vi "gra.vi"() -> ()   [LabVIEW 2016]
doc: "projekt WIiS 201"
panel:
  in  "cluster3":T1
  in  "Cluster 2":T2
  in  "Cluster 1":T3
  out "licznik":i32[][](array[numeric])
  out "obrazy":i32[][](array[ring])
  out "emotikony":u16(ring)
  out "mat17":i32[][](array[numeric])
  out ".not. x?":bool
  out "restart":i32
  out "miny":i32
  out "flag":bool
  out "czas":dbl format="%<%M:%S>t"
  out "miny":i32[][](array[numeric])
  out "rozmiar":i32
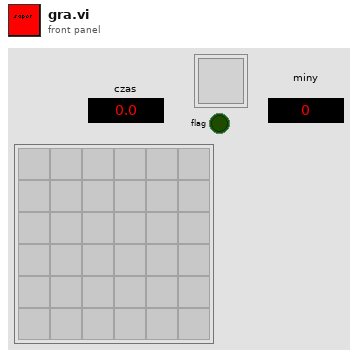
[diagram p1: front panel]
types:
  T1 = cluster{"Boolean 65":bool, "Boolean 66":bool, "Boolean 67":bool, "Boolean 68":bool, "Boolean 69":bool, "Boolean 70":bool, "Boolean 71":bool, "Boolean 72":bool, "Boolean 73":bool, "Boolean 74":bool, "Boolean 75":bool, "Boolean 76":bool, "Boolean 77":bool, "Boolean 78":bool, "Boolean 79":bool, "Boolean 80":bool, "Boolean 81":bool, "Boolean 82":bool, "Boolean 83":bool, "Boolean 84":bool, "Boolean 85":bool, "Boolean 86":bool, "Boolean 87":bool, "Boolean 88":bool, "Boolean 89":bool, "Boolean 90":bool, "Boolean 91":bool, "Boolean 92":bool, "Boolean 93":bool, "Boolean 94":bool, "Boolean 95":bool, "Boolean 96":bool, "Boolean 97":bool, "Boolean 98":bool, "Boolean 99":bool, "Boolean 100":bool, "Boolean 101":bool, "Boolean 102":bool, "Boolean 103":bool, "Boolean 104":bool, "Boolean 105":bool, "Boolean 106":bool, "Boolean 107":bool, "Boolean 108":bool, "Boolean 109":bool, "Boolean 110":bool, "Boolean 111":bool, "Boolean 112":bool, "Boolean 113":bool, "Boolean 114":bool, "Boolean 115":bool, "Boolean 116":bool, "Boolean 117":bool, "Boolean 118":bool, "Boolean 119":bool, "Boolean 120":bool, "Boolean 121":bool, "Boolean 122":bool, "Boolean 123":bool, "Boolean 124":bool, "Boolean 125":bool, "Boolean 126":bool, "Boolean 127":bool, "Boolean 128":bool, "Boolean 129":bool, "Boolean 130":bool, "Boolean 131":bool, "Boolean 132":bool, "Boolean 133":bool, "Boolean 134":bool, "Boolean 135":bool, "Boolean 136":bool, "Boolean 137":bool, "Boolean 138":bool, "Boolean 139":bool, "Boolean 140":bool, "Boolean 141":bool, "Boolean 142":bool, "Boolean 143":bool, "Boolean 144":bool, "Boolean 145":bool, "Boolean 146":bool, "Boolean 147":bool, "Boolean 148":bool, "Boolean 149":bool, "Boolean 150":bool, "Boolean 151":bool, "Boolean 152":bool, "Boolean 153":bool, "Boolean 154":bool, "Boolean 155":bool, "Boolean 156":bool, "Boolean 157":bool, "Boolean 158":bool, "Boolean 159":bool, "Boolean 160":bool, "Boolean 161":bool, "Boolean 162":bool, "Boolean 163":bool, "Boolean 164":bool, "Boolean 165":bool, "Boolean 166":bool, "Boolean 167":bool, "Boolean 168":bool, "Boolean 169":bool, "Boolean 170":bool, "Boolean 171":bool, "Boolean 172":bool, "Boolean 173":bool, "Boolean 174":bool, "Boolean 175":bool, "Boolean 176":bool, "Boolean 177":bool, "Boolean 178":bool, "Boolean 179":bool, "Boolean 180":bool, "Boolean 181":bool, "Boolean 182":bool, "Boolean 183":bool, "Boolean 184":bool, "Boolean 185":bool, "Boolean 186":bool, "Boolean 187":bool, "Boolean 188":bool, "Boolean 189":bool, "Boolean 190":bool, "Boolean 191":bool, "Boolean 192":bool, "Boolean 193":bool, "Boolean 194":bool, "Boolean 195":bool, "Boolean 196":bool, "Boolean 197":bool, "Boolean 198":bool, "Boolean 199":bool, "Boolean 200":bool, "Boolean 201":bool, "Boolean 202":bool, "Boolean 203":bool, "Boolean 204":bool, "Boolean 205":bool, "Boolean 206":bool, "Boolean 207":bool, "Boolean 208":bool}
  T2 = cluster{"Boolean 65":bool, "Boolean 66":bool, "Boolean 67":bool, "Boolean 68":bool, "Boolean 69":bool, "Boolean 70":bool, "Boolean 71":bool, "Boolean 72":bool, "Boolean 77":bool, "Boolean 78":bool, "Boolean 79":bool, "Boolean 80":bool, "Boolean 81":bool, "Boolean 82":bool, "Boolean 83":bool, "Boolean 84":bool, "Boolean 89":bool, "Boolean 90":bool, "Boolean 91":bool, "Boolean 92":bool, "Boolean 93":bool, "Boolean 94":bool, "Boolean 95":bool, "Boolean 96":bool, "Boolean 101":bool, "Boolean 102":bool, "Boolean 103":bool, "Boolean 104":bool, "Boolean 105":bool, "Boolean 106":bool, "Boolean 107":bool, "Boolean 108":bool, "Boolean 113":bool, "Boolean 114":bool, "Boolean 115":bool, "Boolean 116":bool, "Boolean 117":bool, "Boolean 118":bool, "Boolean 119":bool, "Boolean 120":bool, "Boolean 125":bool, "Boolean 126":bool, "Boolean 127":bool, "Boolean 128":bool, "Boolean 129":bool, "Boolean 130":bool, "Boolean 131":bool, "Boolean 132":bool, "Boolean 137":bool, "Boolean 138":bool, "Boolean 139":bool, "Boolean 140":bool, "Boolean 141":bool, "Boolean 142":bool, "Boolean 143":bool, "Boolean 144":bool, "Boolean 149":bool, "Boolean 150":bool, "Boolean 151":bool, "Boolean 152":bool, "Boolean 153":bool, "Boolean 154":bool, "Boolean 155":bool, "Boolean 156":bool}
  T3 = cluster{"Boolean 65":bool, "Boolean 66":bool, "Boolean 67":bool, "Boolean 68":bool, "Boolean 69":bool, "Boolean 70":bool, "Boolean 77":bool, "Boolean 78":bool, "Boolean 79":bool, "Boolean 80":bool, "Boolean 81":bool, "Boolean 82":bool, "Boolean 89":bool, "Boolean 90":bool, "Boolean 91":bool, "Boolean 92":bool, "Boolean 93":bool, "Boolean 94":bool, "Boolean 101":bool, "Boolean 102":bool, "Boolean 103":bool, "Boolean 104":bool, "Boolean 105":bool, "Boolean 106":bool, "Boolean 113":bool, "Boolean 114":bool, "Boolean 115":bool, "Boolean 116":bool, "Boolean 117":bool, "Boolean 118":bool, "Boolean 125":bool, "Boolean 126":bool, "Boolean 127":bool, "Boolean 128":bool, "Boolean 129":bool, "Boolean 130":bool}
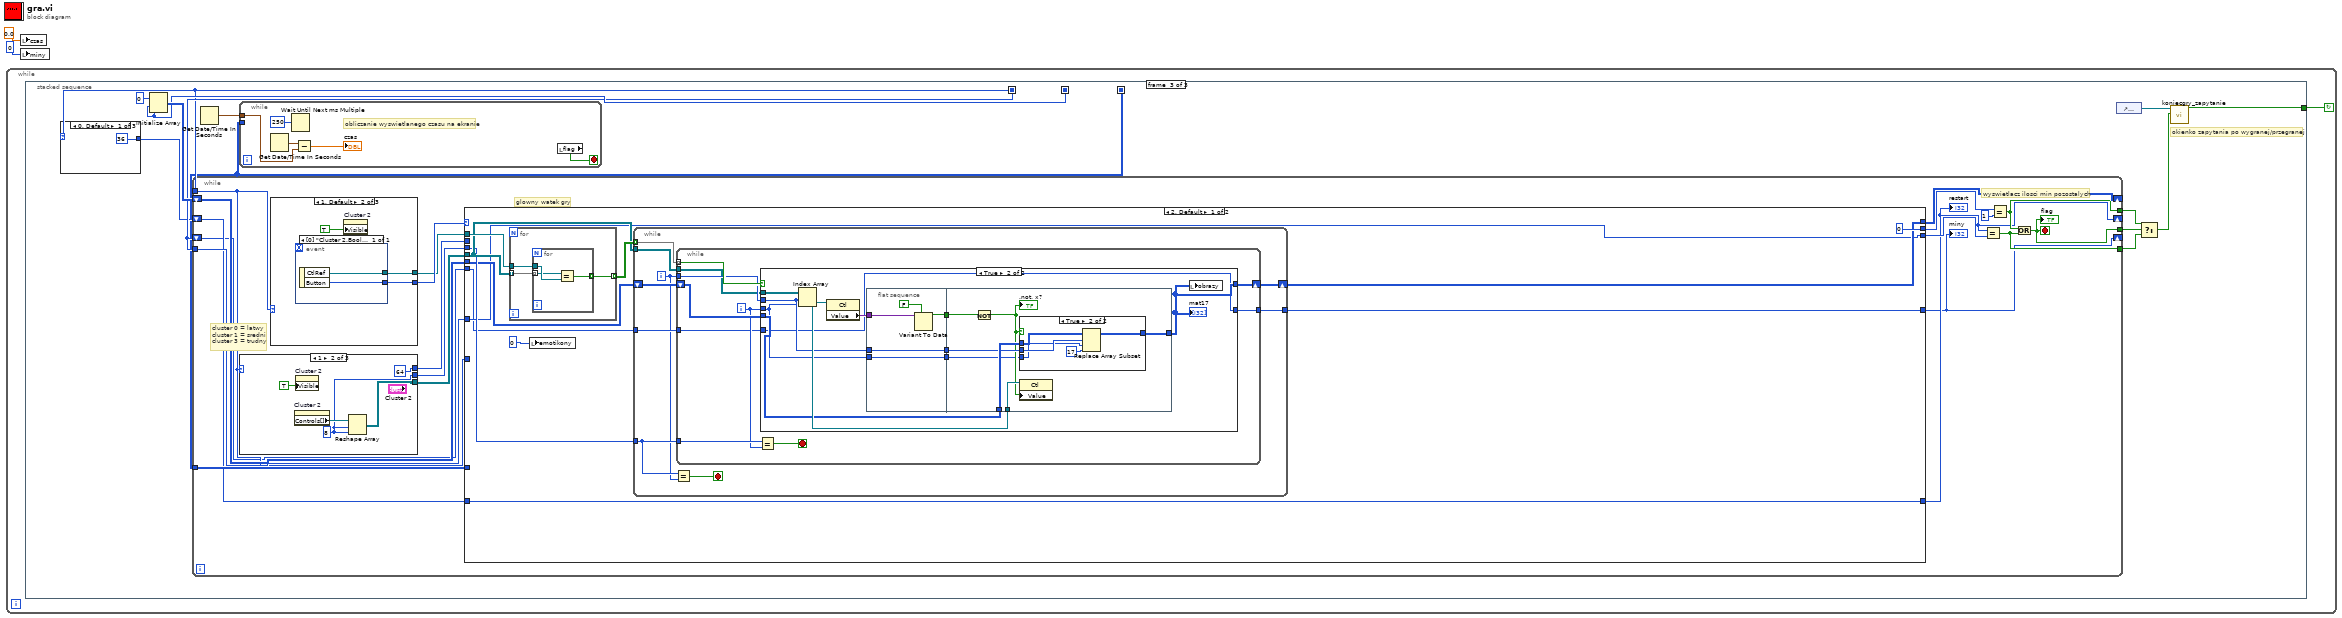
[diagram p0: block diagram]
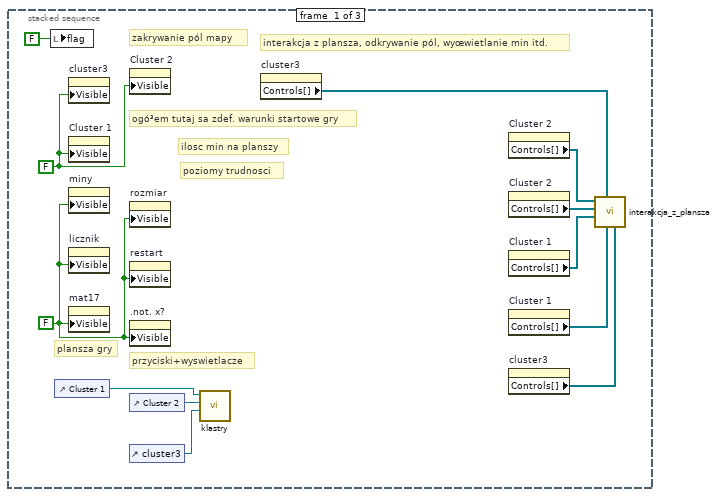
[diagram p2: hidden frame]
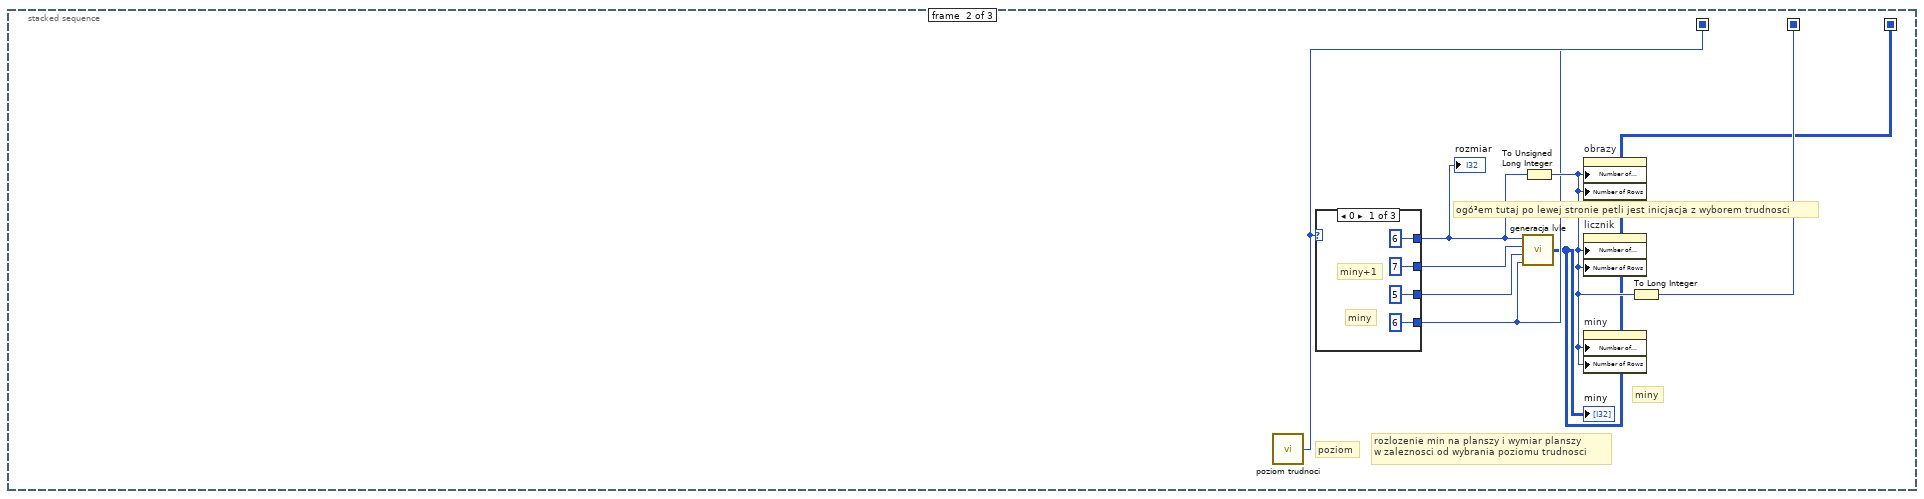
[diagram p3: hidden frame]
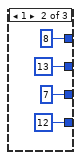
[diagram p4: hidden frame]
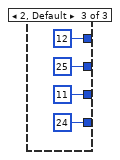
[diagram p5: hidden frame]
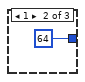
[diagram p6: hidden frame]
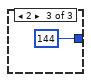
[diagram p7: hidden frame]
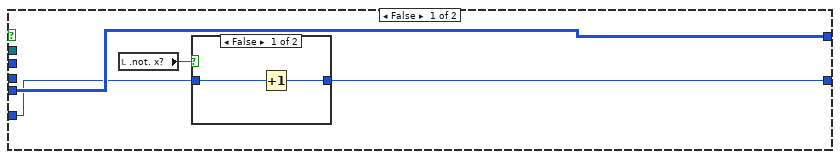
[diagram p8: hidden frame]
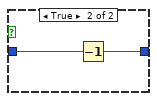
[diagram p9: hidden frame]
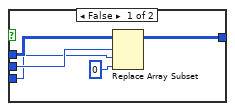
[diagram p10: hidden frame]
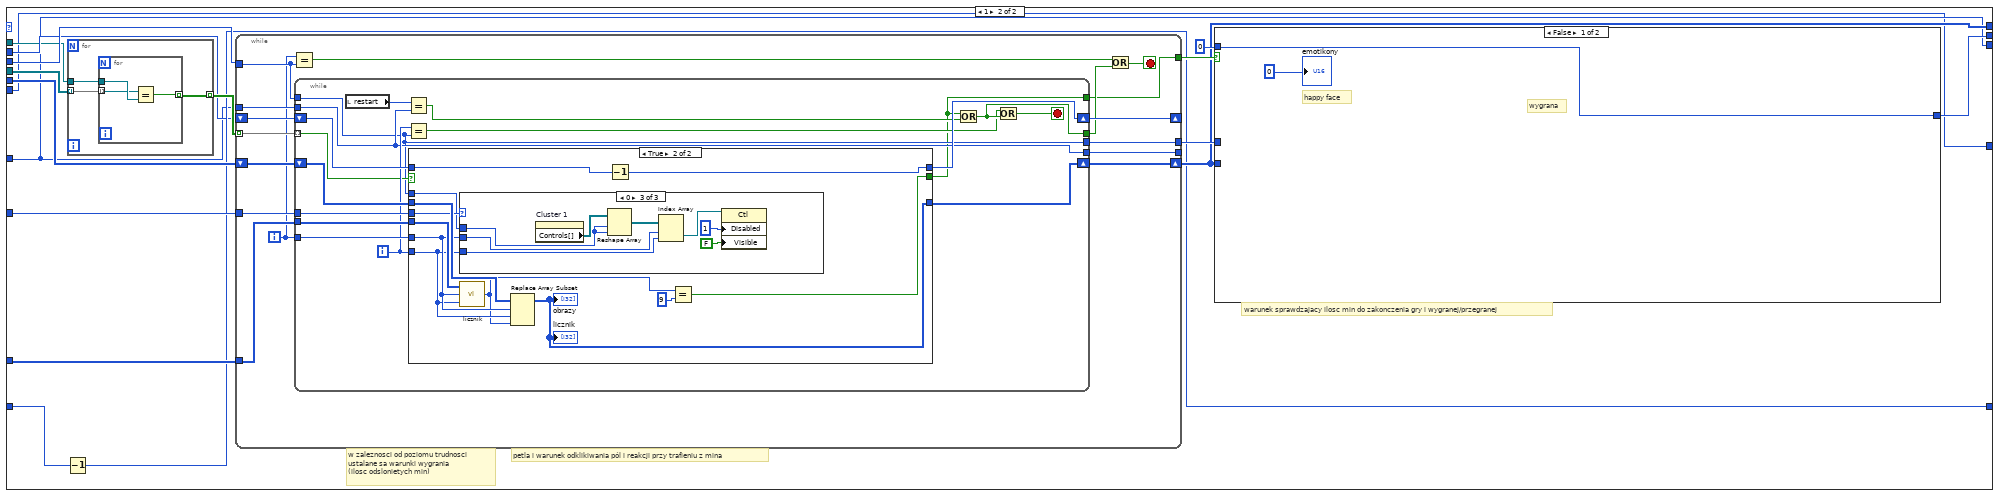
[diagram p11: hidden frame]
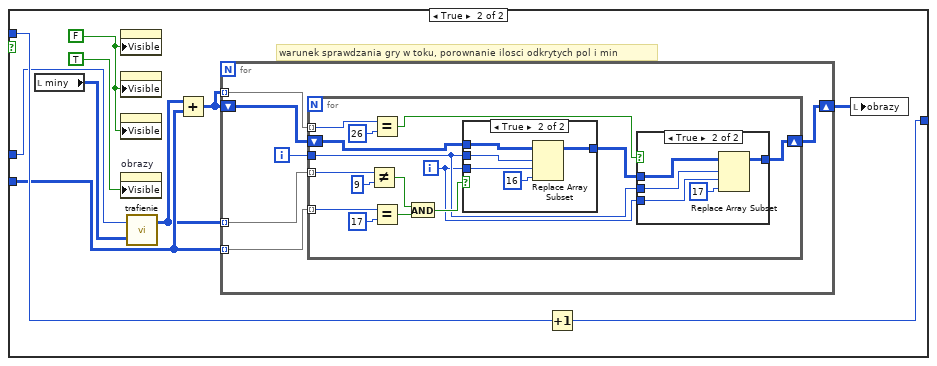
[diagram p12: hidden frame]
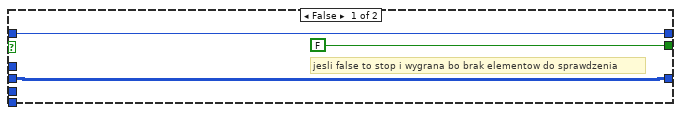
[diagram p15: hidden frame]
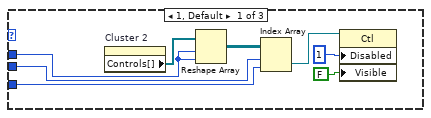
[diagram p16: hidden frame]
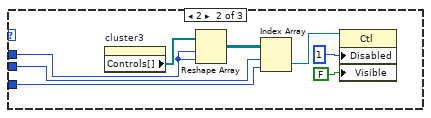
[diagram p17: hidden frame]
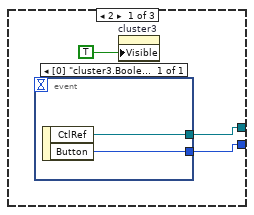
[diagram p18: hidden frame]
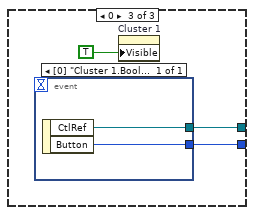
[diagram p19: hidden frame]
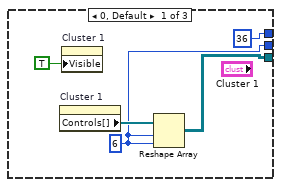
[diagram p20: hidden frame]
diagram:
  n1 = while {
    stop <- w3 continue-if-true
    n2 = stacked-sequence {
      seq-local: [_ w22 _] -> [_ _ w47]
      seq-local: [_ w16 _] -> [_ _ w37]
      seq-local: [_ w20 _] -> [_ _ w43]
      seq-local: [_ w21 _] -> [_ _ w41]
      tunnel: [_ _ w40] -> w3
      frame #0 {
        w8 = FALSE ("Visible")
        w10 = FALSE ("Visible")
        # "przyciski+wyswietlacze"
        # "interakcja z plansza, odkrywanie pól, wyœwietlanie min itd."
        # "ogó³em tutaj sa zdef. warunki startowe gry"
        # "plansza gry"
        # "zakrywanie pól mapy"
        # "ilosc min na planszy"
        # "poziomy trudnosci"
        n3 = local write "flag"(FALSE ("flag")) -> ()
        n4 = control-ref of="Cluster 1"() -> (w6:refnum<vi>)
        n5 = property on="cluster3" class="Clust (strict)"("Visible"=w10) -> ()  [unwired: 2 in, 2 out]
        n6 = property on="Cluster 1" class="Clust (strict)"("Visible"=w10) -> ()  [unwired: 2 in, 2 out]
        n7 = property on="miny" class="Arr (strict)"("Visible"=w8) -> ()  [unwired: 2 in, 2 out]
        n8 = property on="licznik" class="Arr (strict)"("Visible"=w8) -> ()  [unwired: 2 in, 2 out]
        n9 = property on="mat17" class="Arr (strict)"("Visible"=w8) -> ()  [unwired: 2 in, 2 out]
        n10 = property on="Cluster 2" class="Clust (strict)"("Visible"=w10) -> ()  [unwired: 2 in, 2 out]
        n11 = property on="rozmiar" class="DigNum (strict)"("Visible"=w8) -> ()  [unwired: 2 in, 2 out]
        n12 = property on="restart" class="DigNum (strict)"("Visible"=w8) -> ()  [unwired: 2 in, 2 out]
        n13 = property on=".not. x?" class="Bool (strict)"("Visible"=w8) -> ()  [unwired: 2 in, 2 out]
        n14 = control-ref of="Cluster 2"() -> (w5:refnum<vi>)
        n15 = control-ref of="cluster3"() -> (w4:refnum<vi>)
        n16 = call "klastry.vi"("reference 3"=w4, "reference in"=w5, "Cluster in"=w6) -> ()  [unwired: 9 in]
        n17 = property on="cluster3" class="Clust (strict)"() -> ("Controls[]"=w12:refnum<vi>[])  [unwired: 2 in, 2 out]
        n18 = property on="Cluster 2" class="Clust (strict)"() -> ("Controls[]"=w14:refnum<vi>[])  [unwired: 2 in, 2 out]
        n19 = property on="Cluster 2" class="Clust (strict)"() -> ("Controls[]"=w11:refnum<vi>[])  [unwired: 2 in, 2 out]
        n20 = property on="Cluster 1" class="Clust (strict)"() -> ("Controls[]"=w9:refnum<vi>[])  [unwired: 2 in, 2 out]
        n21 = property on="Cluster 1" class="Clust (strict)"() -> ("Controls[]"=w15:refnum<vi>[])  [unwired: 2 in, 2 out]
        n22 = property on="cluster3" class="Clust (strict)"() -> ("Controls[]"=w13:refnum<vi>[])  [unwired: 2 in, 2 out]
        n23 = call "interakcja_z_plansza.vi"("Controls[] 4"=w13, "Controls[] 6"=w15, "Controls[] 3"=w12, "Controls[]"=w9, "Controls[] 2"=w11, "Controls[] 5"=w14) -> ()  [unwired: 6 in]
      }
      frame #1 {
        # "ogó³em tutaj po lewej stronie petli jest inicjacja z wyborem trudnosci"
        # "miny"
        # "poziom"
        # "rozlozenie min na planszy i wymiar planszy \nw zaleznosci od wybrania poziomu trudnosci"
        n24 = call "poziom trudnoci.vi"() -> ("wynik wyboru"=w21:i32)
        n25 = case shown="0" w21 {
          tunnel: [6 8 12] -> w17
          tunnel: [7 13 25] -> w18
          tunnel: [6 12 24] -> w20
          tunnel: [5 7 11] -> w19
          frame 0 {
            # "miny"
            # "miny+1"
          }
          frame 1 {
          }
          frame 2, Default {
          }
        }
        "rozmiar" <- w17
        n26 = call "generacja lvle.vi"("miny"=w20, "const"=w19, "Miny+1"=w18, "rozmiar"=w17) -> ("Array"=w16:i32[][])
        "miny" <- w16
        n27 = To Unsigned Long Integer(number=w17) -> (unsigned 32bit integer=w23:u32)
        n28 = property on="obrazy" class="Arr (strict)"("Number of Columns"=w23, "Number of Rows"=w23) -> ()  [unwired: 2 in, 2 out]
        n29 = property on="licznik" class="Arr (strict)"("Number of Columns"=w23, "Number of Rows"=w23) -> ()  [unwired: 2 in, 2 out]
        n30 = property on="miny" class="Arr (strict)"("Number of Columns"=w23, "Number of Rows"=w23) -> ()  [unwired: 2 in, 2 out]
        n31 = To Long Integer(number=w23) -> (32bit integer=w22:i32)
      }
      frame #2 {
        # "okienko zapytania po wygranej/przegranej"
        n32 = case shown="0, Default" w41 {
          tunnel: [36 ("dimension size") 64 ("dimension size") 144 ("dimension size")] -> w42
          frame 0, Default {
          }
          frame 1 {
          }
          frame 2 {
          }
        }
        n33 = Initialize Array(0 ("element"), w47, w47) -> (w48:i32[][])
        n34 = while {
          tunnel: w37 -> [w77]
          tunnel: w41 -> [w69]
          shift-right: [w67] -> _
          shift-left: w48 -> [w76]
          tunnel: w43 -> [w74]
          tunnel: [w61] -> w39
          tunnel: [w62] -> w46
          tunnel: [w63] -> w45
          shift-right: [w60] -> _
          shift-left: w42 -> [w65]
          shift-right: [w58] -> _
          shift-left: w43 -> [w59]
          stop <- w61 stop-if-true
          # "cluster 0 = latwy\ncluster 1 = sredni\ncluster 3 = trudny"
          # "glowny watek gry"
          # "wyswietlacz ilosci min pozostalych"
          n35 = case shown="1" w69 {
            tunnel: [w312 w317 w322] -> w75
            tunnel: [36 ("dimension size") 64 ("element") 144] -> w73
            tunnel: [w311 w316 w321] -> w68
            frame 0, Default {
              w312 = 6 ("dimension size")
              n36 = property on="Cluster 1" class="Clust (strict)"() -> ("Controls[]"=w313:refnum<vi>[])  [unwired: 2 in, 2 out]
              n37 = property on="Cluster 1" class="Clust (strict)"("Visible"=TRUE) -> ()  [unwired: 2 in, 2 out]
              n38 = Reshape Array(w313, w312, w312) -> (w311:refnum<vi>[][])
            }
            frame 1 {
              w317 = 8 ("element")
              n39 = property on="Cluster 2" class="Clust (strict)"() -> ("Controls[]"=w318:refnum<vi>[])  [unwired: 2 in, 2 out]
              n40 = property on="Cluster 2" class="Clust (strict)"("Visible"=TRUE) -> ()  [unwired: 2 in, 2 out]
              n41 = Reshape Array(w318, w317, w317) -> (w316:refnum<vi>[][])
            }
            frame 2 {
              w322 = 12 ("element")
              n42 = property on="cluster3" class="Clust (strict)"("Visible"=TRUE) -> ()  [unwired: 2 in, 2 out]
              n43 = property on="cluster3" class="Clust (strict)"() -> ("Controls[]"=w323:refnum<vi>[])  [unwired: 2 in, 2 out]
              n44 = Reshape Array(w323, w322, w322) -> (w321:refnum<vi>[][])
            }
          }
          n45 = case shown="1, Default" w69 {
            tunnel: [w298 w303 w308] -> w71
            tunnel: [w297 w302 w306] -> w70
            frame 2 {
              n46 = event shown="[0] \"cluster3.Boolean 65\", \"cluster3.Boolean 66\", \"cluster3.Boolean 67\", \"cluster3.Boolean 68\", \"cluster3.Boolean 69\", \"cluster3.Boolean 70\", \"cluster3.Boolean 71\", \"cluster3.Boolean 72\", \"cluster3.Boolean 73\", \"cluster3.Boolean 74\", \"cluster3.Boolean 75\", \"cluster3.Boolean 76\", \"cluster3.Boolean 77\", \"cluster3.Boolean 78\", \"cluster3.Boolean 79\", \"cluster3.Boolean 80\", \"cluster3.Boolean 81\", \"cluster3.Boolean 82\", \"cluster3.Boolean 83\", \"cluster3.Boolean 84\", \"cluster3.Boolean 85\", \"cluster3.Boolean 86\", \"cluster3.Boolean 87\", \"cluster3.Boolean 88\", \"cluster3.Boolean 89\", \"cluster3.Boolean 90\", \"cluster3.Boolean 91\", \"cluster3.Boolean 92\", \"cluster3.Boolean 93\", \"cluster3.Boolean 94\", \"cluster3.Boolean 95\", \"cluster3.Boolean 96\", \"cluster3.Boolean 97\", \"cluster3.Boolean 98\", \"cluster3.Boolean 99\", \"cluster3.Boolean 100\", \"cluster3.Boolean 101\", \"cluster3.Boolean 102\", \"cluster3.Boolean 103\", \"cluster3.Boolean 104\", \"cluster3.Boolean 105\", \"cluster3.Boolean 106\", \"cluster3.Boolean 107\", \"cluster3.Boolean 108\", \"cluster3.Boolean 109\", \"cluster3.Boolean 110\", \"cluster3.Boolean 111\", \"cluster3.Boolean 112\", \"cluster3.Boolean 113\", \"cluster3.Boolean 114\", \"cluster3.Boolean 115\", \"cluster3.Boolean 116\", \"cluster3.Boolean 117\", \"cluster3.Boolean 118\", \"cluster3.Boolean 119\", \"cluster3.Boolean 120\", \"cluster3.Boolean 121\", \"cluster3.Boolean 122\", \"cluster3.Boolean 123\", \"cluster3.Boolean 124\", \"cluster3.Boolean 125\", \"cluster3.Boolean 126\", \"cluster3.Boolean 127\", \"cluster3.Boolean 128\", \"cluster3.Boolean 129\", \"cluster3.Boolean 130\", \"cluster3.Boolean 131\", \"cluster3.Boolean 132\", \"cluster3.Boolean 133\", \"cluster3.Boolean 134\", \"cluster3.Boolean 135\", \"cluster3.Boolean 136\", \"cluster3.Boolean 137\", \"cluster3.Boolean 138\", \"cluster3.Boolean 139\", \"cluster3.Boolean 140\", \"cluster3.Boolean 141\", \"cluster3.Boolean 142\", \"cluster3.Boolean 143\", \"cluster3.Boolean 144\", \"cluster3.Boolean 145\", \"cluster3.Boolean 146\", \"cluster3.Boolean 147\", \"cluster3.Boolean 148\", \"cluster3.Boolean 149\", \"cluster3.Boolean 150\", \"cluster3.Boolean 151\", \"cluster3.Boolean 152\", \"cluster3.Boolean 153\", \"cluster3.Boolean 154\", \"cluster3.Boolean 155\", \"cluster3.Boolean 156\", \"cluster3.Boolean 157\", \"cluster3.Boolean 158\", \"cluster3.Boolean 159\", \"cluster3.Boolean 160\", \"cluster3.Boolean 161\", \"cluster3.Boolean 162\", \"cluster3.Boolean 163\", \"cluster3.Boolean 164\", \"cluster3.Boolean 165\", \"cluster3.Boolean 166\", \"cluster3.Boolean 167\", \"cluster3.Boolean 168\", \"cluster3.Boolean 169\", \"cluster3.Boolean 170\", \"cluster3.Boolean 171\", \"cluster3.Boolean 172\", \"cluster3.Boolean 173\", \"cluster3.Boolean 174\", \"cluster3.Boolean 175\", \"cluster3.Boolean 176\", \"cluster3.Boolean 177\", \"cluster3.Boolean 178\", \"cluster3.Boolean 179\", \"cluster3.Boolean 180\", \"cluster3.Boolean 181\", \"cluster3.Boolean 182\", \"cluster3.Boolean 183\", \"cluster3.Boolean 184\", \"cluster3.Boolean 185\", \"cluster3.Boolean 186\", \"cluster3.Boolean 187\", \"cluster3.Boolean 188\", \"cluster3.Boolean 189\", \"cluster3.Boolean 190\", \"cluster3.Boolean 191\", \"cluster3.Boolean 192\", \"cluster3.Boolean 193\", \"cluster3.Boolean 194\", \"cluster3.Boolean 195\", \"cluster3.Boolean 196\", \"cluster3.Boolean 197\", \"cluster3.Boolean 198\", \"cluster3.Boolean 199\", \"cluster3.Boolean 200\", \"cluster3.Boolean 201\", \"cluster3.Boolean 202\", \"cluster3.Boolean 203\", \"cluster3.Boolean 204\", \"cluster3.Boolean 205\", \"cluster3.Boolean 206\", \"cluster3.Boolean 207\", \"cluster3.Boolean 208\": Mouse Down" {
                selector: _ -> [_]
                dyn-events: _ -> [_]
                timeout: _ -> [_]
                tunnel: [w299] -> w298
                tunnel: [w300] -> w297
                event "cluster3.Boolean 65", "cluster3.Boolean 66", "cluster3.Boolean 67", "cluster3.Boolean 68", "cluster3.Boolean 69", "cluster3.Boolean 70", "cluster3.Boolean 71", "cluster3.Boolean 72", "cluster3.Boolean 73", "cluster3.Boolean 74", "cluster3.Boolean 75", "cluster3.Boolean 76", "cluster3.Boolean 77", "cluster3.Boolean 78", "cluster3.Boolean 79", "cluster3.Boolean 80", "cluster3.Boolean 81", "cluster3.Boolean 82", "cluster3.Boolean 83", "cluster3.Boolean 84", "cluster3.Boolean 85", "cluster3.Boolean 86", "cluster3.Boolean 87", "cluster3.Boolean 88", "cluster3.Boolean 89", "cluster3.Boolean 90", "cluster3.Boolean 91", "cluster3.Boolean 92", "cluster3.Boolean 93", "cluster3.Boolean 94", "cluster3.Boolean 95", "cluster3.Boolean 96", "cluster3.Boolean 97", "cluster3.Boolean 98", "cluster3.Boolean 99", "cluster3.Boolean 100", "cluster3.Boolean 101", "cluster3.Boolean 102", "cluster3.Boolean 103", "cluster3.Boolean 104", "cluster3.Boolean 105", "cluster3.Boolean 106", "cluster3.Boolean 107", "cluster3.Boolean 108", "cluster3.Boolean 109", "cluster3.Boolean 110", "cluster3.Boolean 111", "cluster3.Boolean 112", "cluster3.Boolean 113", "cluster3.Boolean 114", "cluster3.Boolean 115", "cluster3.Boolean 116", "cluster3.Boolean 117", "cluster3.Boolean 118", "cluster3.Boolean 119", "cluster3.Boolean 120", "cluster3.Boolean 121", "cluster3.Boolean 122", "cluster3.Boolean 123", "cluster3.Boolean 124", "cluster3.Boolean 125", "cluster3.Boolean 126", "cluster3.Boolean 127", "cluster3.Boolean 128", "cluster3.Boolean 129", "cluster3.Boolean 130", "cluster3.Boolean 131", "cluster3.Boolean 132", "cluster3.Boolean 133", "cluster3.Boolean 134", "cluster3.Boolean 135", "cluster3.Boolean 136", "cluster3.Boolean 137", "cluster3.Boolean 138", "cluster3.Boolean 139", "cluster3.Boolean 140", "cluster3.Boolean 141", "cluster3.Boolean 142", "cluster3.Boolean 143", "cluster3.Boolean 144", "cluster3.Boolean 145", "cluster3.Boolean 146", "cluster3.Boolean 147", "cluster3.Boolean 148", "cluster3.Boolean 149", "cluster3.Boolean 150", "cluster3.Boolean 151", "cluster3.Boolean 152", "cluster3.Boolean 153", "cluster3.Boolean 154", "cluster3.Boolean 155", "cluster3.Boolean 156", "cluster3.Boolean 157", "cluster3.Boolean 158", "cluster3.Boolean 159", "cluster3.Boolean 160", "cluster3.Boolean 161", "cluster3.Boolean 162", "cluster3.Boolean 163", "cluster3.Boolean 164", "cluster3.Boolean 165", "cluster3.Boolean 166", "cluster3.Boolean 167", "cluster3.Boolean 168", "cluster3.Boolean 169", "cluster3.Boolean 170", "cluster3.Boolean 171", "cluster3.Boolean 172", "cluster3.Boolean 173", "cluster3.Boolean 174", "cluster3.Boolean 175", "cluster3.Boolean 176", "cluster3.Boolean 177", "cluster3.Boolean 178", "cluster3.Boolean 179", "cluster3.Boolean 180", "cluster3.Boolean 181", "cluster3.Boolean 182", "cluster3.Boolean 183", "cluster3.Boolean 184", "cluster3.Boolean 185", "cluster3.Boolean 186", "cluster3.Boolean 187", "cluster3.Boolean 188", "cluster3.Boolean 189", "cluster3.Boolean 190", "cluster3.Boolean 191", "cluster3.Boolean 192", "cluster3.Boolean 193", "cluster3.Boolean 194", "cluster3.Boolean 195", "cluster3.Boolean 196", "cluster3.Boolean 197", "cluster3.Boolean 198", "cluster3.Boolean 199", "cluster3.Boolean 200", "cluster3.Boolean 201", "cluster3.Boolean 202", "cluster3.Boolean 203", "cluster3.Boolean 204", "cluster3.Boolean 205", "cluster3.Boolean 206", "cluster3.Boolean 207", "cluster3.Boolean 208": Mouse Down {
                  n47 = event-data() -> ("CtlRef"=w300:refnum<vi>, "Button"=w299:u16)  [unwired: 1 in]
                }
              }
              n48 = property on="cluster3" class="Clust (strict)"("Visible"=TRUE) -> ()  [unwired: 2 in, 2 out]
            }
            frame 1, Default {
              n49 = event shown="[0] \"Cluster 2.Boolean 65\", \"Cluster 2.Boolean 66\", \"Cluster 2.Boolean 67\", \"Cluster 2.Boolean 68\", \"Cluster 2.Boolean 69\", \"Cluster 2.Boolean 70\", \"Cluster 2.Boolean 71\", \"Cluster 2.Boolean 72\", \"Cluster 2.Boolean 77\", \"Cluster 2.Boolean 78\", \"Cluster 2.Boolean 79\", \"Cluster 2.Boolean 80\", \"Cluster 2.Boolean 81\", \"Cluster 2.Boolean 82\", \"Cluster 2.Boolean 83\", \"Cluster 2.Boolean 84\", \"Cluster 2.Boolean 89\", \"Cluster 2.Boolean 90\", \"Cluster 2.Boolean 91\", \"Cluster 2.Boolean 92\", \"Cluster 2.Boolean 93\", \"Cluster 2.Boolean 94\", \"Cluster 2.Boolean 95\", \"Cluster 2.Boolean 96\", \"Cluster 2.Boolean 101\", \"Cluster 2.Boolean 102\", \"Cluster 2.Boolean 103\", \"Cluster 2.Boolean 104\", \"Cluster 2.Boolean 105\", \"Cluster 2.Boolean 106\", \"Cluster 2.Boolean 107\", \"Cluster 2.Boolean 108\", \"Cluster 2.Boolean 113\", \"Cluster 2.Boolean 114\", \"Cluster 2.Boolean 115\", \"Cluster 2.Boolean 116\", \"Cluster 2.Boolean 117\", \"Cluster 2.Boolean 118\", \"Cluster 2.Boolean 119\", \"Cluster 2.Boolean 120\", \"Cluster 2.Boolean 125\", \"Cluster 2.Boolean 126\", \"Cluster 2.Boolean 127\", \"Cluster 2.Boolean 128\", \"Cluster 2.Boolean 129\", \"Cluster 2.Boolean 130\", \"Cluster 2.Boolean 131\", \"Cluster 2.Boolean 132\", \"Cluster 2.Boolean 137\", \"Cluster 2.Boolean 138\", \"Cluster 2.Boolean 139\", \"Cluster 2.Boolean 140\", \"Cluster 2.Boolean 141\", \"Cluster 2.Boolean 142\", \"Cluster 2.Boolean 143\", \"Cluster 2.Boolean 144\", \"Cluster 2.Boolean 149\", \"Cluster 2.Boolean 150\", \"Cluster 2.Boolean 151\", \"Cluster 2.Boolean 152\", \"Cluster 2.Boolean 153\", \"Cluster 2.Boolean 154\", \"Cluster 2.Boolean 155\", \"Cluster 2.Boolean 156\": Mouse Down" {
                selector: _ -> [_]
                dyn-events: _ -> [_]
                timeout: _ -> [_]
                tunnel: [w305] -> w303
                tunnel: [w304] -> w302
                event "Cluster 2.Boolean 65", "Cluster 2.Boolean 66", "Cluster 2.Boolean 67", "Cluster 2.Boolean 68", "Cluster 2.Boolean 69", "Cluster 2.Boolean 70", "Cluster 2.Boolean 71", "Cluster 2.Boolean 72", "Cluster 2.Boolean 77", "Cluster 2.Boolean 78", "Cluster 2.Boolean 79", "Cluster 2.Boolean 80", "Cluster 2.Boolean 81", "Cluster 2.Boolean 82", "Cluster 2.Boolean 83", "Cluster 2.Boolean 84", "Cluster 2.Boolean 89", "Cluster 2.Boolean 90", "Cluster 2.Boolean 91", "Cluster 2.Boolean 92", "Cluster 2.Boolean 93", "Cluster 2.Boolean 94", "Cluster 2.Boolean 95", "Cluster 2.Boolean 96", "Cluster 2.Boolean 101", "Cluster 2.Boolean 102", "Cluster 2.Boolean 103", "Cluster 2.Boolean 104", "Cluster 2.Boolean 105", "Cluster 2.Boolean 106", "Cluster 2.Boolean 107", "Cluster 2.Boolean 108", "Cluster 2.Boolean 113", "Cluster 2.Boolean 114", "Cluster 2.Boolean 115", "Cluster 2.Boolean 116", "Cluster 2.Boolean 117", "Cluster 2.Boolean 118", "Cluster 2.Boolean 119", "Cluster 2.Boolean 120", "Cluster 2.Boolean 125", "Cluster 2.Boolean 126", "Cluster 2.Boolean 127", "Cluster 2.Boolean 128", "Cluster 2.Boolean 129", "Cluster 2.Boolean 130", "Cluster 2.Boolean 131", "Cluster 2.Boolean 132", "Cluster 2.Boolean 137", "Cluster 2.Boolean 138", "Cluster 2.Boolean 139", "Cluster 2.Boolean 140", "Cluster 2.Boolean 141", "Cluster 2.Boolean 142", "Cluster 2.Boolean 143", "Cluster 2.Boolean 144", "Cluster 2.Boolean 149", "Cluster 2.Boolean 150", "Cluster 2.Boolean 151", "Cluster 2.Boolean 152", "Cluster 2.Boolean 153", "Cluster 2.Boolean 154", "Cluster 2.Boolean 155", "Cluster 2.Boolean 156": Mouse Down {
                  n50 = event-data() -> ("CtlRef"=w304:refnum<vi>, "Button"=w305:u16)  [unwired: 1 in]
                }
              }
              n51 = property on="Cluster 2" class="Clust (strict)"("Visible"=TRUE) -> ()  [unwired: 2 in, 2 out]
            }
            frame 0 {
              n52 = event shown="[0] \"Cluster 1.Boolean 65\", \"Cluster 1.Boolean 66\", \"Cluster 1.Boolean 67\", \"Cluster 1.Boolean 68\", \"Cluster 1.Boolean 69\", \"Cluster 1.Boolean 70\", \"Cluster 1.Boolean 77\", \"Cluster 1.Boolean 78\", \"Cluster 1.Boolean 80\", \"Cluster 1.Boolean 79\", \"Cluster 1.Boolean 81\", \"Cluster 1.Boolean 82\", \"Cluster 1.Boolean 89\", \"Cluster 1.Boolean 90\", \"Cluster 1.Boolean 91\", \"Cluster 1.Boolean 92\", \"Cluster 1.Boolean 93\", \"Cluster 1.Boolean 94\", \"Cluster 1.Boolean 101\", \"Cluster 1.Boolean 102\", \"Cluster 1.Boolean 103\", \"Cluster 1.Boolean 104\", \"Cluster 1.Boolean 105\", \"Cluster 1.Boolean 106\", \"Cluster 1.Boolean 113\", \"Cluster 1.Boolean 114\", \"Cluster 1.Boolean 115\", \"Cluster 1.Boolean 116\", \"Cluster 1.Boolean 117\", \"Cluster 1.Boolean 118\", \"Cluster 1.Boolean 125\", \"Cluster 1.Boolean 126\", \"Cluster 1.Boolean 127\", \"Cluster 1.Boolean 128\", \"Cluster 1.Boolean 129\", \"Cluster 1.Boolean 130\": Mouse Down" {
                selector: _ -> [_]
                dyn-events: _ -> [_]
                timeout: _ -> [_]
                tunnel: [w309] -> w308
                tunnel: [w310] -> w306
                event "Cluster 1.Boolean 65", "Cluster 1.Boolean 66", "Cluster 1.Boolean 67", "Cluster 1.Boolean 68", "Cluster 1.Boolean 69", "Cluster 1.Boolean 70", "Cluster 1.Boolean 77", "Cluster 1.Boolean 78", "Cluster 1.Boolean 80", "Cluster 1.Boolean 79", "Cluster 1.Boolean 81", "Cluster 1.Boolean 82", "Cluster 1.Boolean 89", "Cluster 1.Boolean 90", "Cluster 1.Boolean 91", "Cluster 1.Boolean 92", "Cluster 1.Boolean 93", "Cluster 1.Boolean 94", "Cluster 1.Boolean 101", "Cluster 1.Boolean 102", "Cluster 1.Boolean 103", "Cluster 1.Boolean 104", "Cluster 1.Boolean 105", "Cluster 1.Boolean 106", "Cluster 1.Boolean 113", "Cluster 1.Boolean 114", "Cluster 1.Boolean 115", "Cluster 1.Boolean 116", "Cluster 1.Boolean 117", "Cluster 1.Boolean 118", "Cluster 1.Boolean 125", "Cluster 1.Boolean 126", "Cluster 1.Boolean 127", "Cluster 1.Boolean 128", "Cluster 1.Boolean 129", "Cluster 1.Boolean 130": Mouse Down {
                  n53 = event-data() -> ("CtlRef"=w310:refnum<vi>, "Button"=w309:u16)  [unwired: 1 in]
                }
              }
              n54 = property on="Cluster 1" class="Clust (strict)"("Visible"=TRUE) -> ()  [unwired: 2 in, 2 out]
            }
          }
          n55 = case shown="2, Default" w71 {
            tunnel: w77 -> [_ w172]
            tunnel: w69 -> [_ w171]
            tunnel: w76 -> [w84 w170]
            tunnel: [w83 w163] -> w67
            tunnel: w75 -> [w85 w169]
            tunnel: w74 -> [w80 w157]
            tunnel: [0 w166] -> w66
            tunnel: w73 -> [_ w161]
            tunnel: w70 -> [w89 w159]
            tunnel: w68 -> [w87 w160]
            tunnel: [w80 w157] -> w64
            tunnel: [w82 w162] -> w60
            tunnel: w65 -> [w82 w158]
            tunnel: [w78 w156] -> w58
            tunnel: w59 -> [w79 w156]
            frame 2, Default {
              n56 = for {
                tunnel: w89 -> [w152]
                tunnel: w87 -> [w151] mode=indexing
                tunnel: [w150] -> w88 mode=indexing
                n57 = for {
                  tunnel: w152 -> [w155]
                  tunnel: w151 -> [w154] mode=indexing
                  tunnel: [w153] -> w150 mode=indexing
                  n58 = Equal?(x=w154, y=w155) -> (x = y?=w153:bool)
                }
              }
              n59 = local write "emotikony"(u16 0 ("caras 2")) -> ()
              n60 = while {
                tunnel: w88 -> [w98] mode=indexing
                shift-right: [w93] -> w83
                shift-left: w84 -> [w97]
                tunnel: w87 -> [w96]
                tunnel: w85 -> [w95]
                tunnel: w79 -> [w92]
                tunnel: [w90] -> w78
                i -> [w91]
                stop <- w94 stop-if-true
                n61 = Equal?(x=w95, y=w91) -> (x = y?=w94:bool)
                n62 = while {
                  tunnel: w98 -> [w108] mode=indexing
                  tunnel: w91 -> [w106]
                  shift-right: [w105] -> w93
                  shift-left: w97 -> [w107]
                  tunnel: w96 -> [w104]
                  tunnel: w95 -> [w103]
                  tunnel: w92 -> [w101]
                  tunnel: [w100] -> w90
                  i -> [w102]
                  stop <- w99 stop-if-true
                  n63 = Equal?(x=w103, y=w102) -> (x = y?=w99:bool)
                  n64 = case shown="True" w108 {
                    tunnel: w107 -> [w112 w123]
                    tunnel: w106 -> [_ w121]
                    tunnel: [w112 w120] -> w105
                    tunnel: w104 -> [_ w127]
                    tunnel: w102 -> [_ w118]
                    tunnel: w101 -> [w110 w117]
                    tunnel: [w109 w117] -> w100
                    frame False {
                      n65 = local read ".not. x?"() -> (w111:bool)
                      n66 = case shown="False" w111 {
                        tunnel: [w114 w116] -> w109
                        tunnel: w110 -> [w113 w115]
                        frame False {
                          n67 = Increment(x=w113) -> (x+1=w114:i32)
                        }
                        frame True {
                          n68 = Decrement(x=w115) -> (x-1=w116:i32)
                        }
                      }
                    }
                    frame True {
                      n69 = Index Array(array=w127, index (row)=w121, index (col)=w118) -> (element=w124:refnum<vi>)
                      n70 = property class="Ctl"(reference=w124) -> ("Value"=w125:variant)  [unwired: 1 in, 2 out]
                      n71 = flat-sequence {
                        tunnel: w125 -> [w132]
                        tunnel: [w128] -> w126
                        tunnel: [w131] -> w122
                        tunnel: w121 -> [w131]
                        tunnel: w118 -> [w129]
                        tunnel: [w129] -> w119
                        tunnel: w126 -> [w139]
                        tunnel: w124 -> [w138]
                        tunnel: w123 -> [w137]
                        tunnel: w122 -> [w136]
                        tunnel: [w135] -> w120
                        tunnel: w119 -> [w133]
                        frame #0 {
                          n72 = Variant To Data(type=FALSE ("Visible"), Variant=w132) -> (data=w128:bool)  [unwired: 1 in, 1 out]
                        }
                        frame #1 {
                          n73 = Not(x=w139) -> (.not. x?=w134:bool)
                          ".not. x?" <- w134
                          n74 = case shown="True" w134 {
                            tunnel: w137 -> [w144 w149]
                            tunnel: w136 -> [w142 w148]
                            tunnel: [w143 w146] -> w135
                            tunnel: w133 -> [w140 w147]
                            frame False {
                              n75 = Replace Array Subset(array=w144, new element=0 ("new element/subarray"), index (row)=w142, index (col)=w140) -> (w143:i32[][])
                            }
                            frame True {
                              n76 = Replace Array Subset(array=w149, new element=17 ("new element/subarray"), index (row)=w148, index (col)=w147) -> (w146:i32[][])
                            }
                          }
                          n77 = property class="Ctl"(reference=w138, "Value"=w134) -> ()  [unwired: 1 in, 2 out]
                        }
                      }
                      n78 = local write "obrazy"(w120) -> ()
                      "mat17" <- w120
                    }
                  }
                }
              }
            }
            frame 1 {
              # "w zaleznosci od poziomu trudnosci\nustalane sa warunki wygrania\n(ilosc odslonietych min)"
              # "petla i warunek odklikiwania pól i reakcji przy trafieniu z mina"
              # "warunek sprawdzajacy ilosc min do zakonczenia gry i wygranej/przegranej"
              n79 = Decrement(x=w158) -> (x-1=w162:i32)
              n80 = for {
                tunnel: w159 -> [w175]
                tunnel: [w174] -> w164 mode=indexing
                tunnel: w160 -> [w173] mode=indexing
                n81 = for {
                  tunnel: w173 -> [w176] mode=indexing
                  tunnel: w175 -> [w178]
                  tunnel: [w177] -> w174 mode=indexing
                  n82 = Equal?(x=w176, y=w178) -> (x = y?=w177:bool)
                }
              }
              n83 = while {
                shift-right: [w238] -> w163
                shift-left: w170 -> [w239]
                tunnel: w172 -> [w237]
                tunnel: w169 -> [w231]
                tunnel: w171 -> [w236]
                tunnel: w157 -> [w235]
                shift-right: [w232] -> _
                shift-left: w161 -> [w234]
                tunnel: [w233] -> _
                tunnel: [w227] -> w168
                tunnel: [w226] -> w167
                tunnel: w164 -> [w225] mode=indexing
                i -> [w224]
                stop <- w229 stop-if-true
                n84 = Equal?(x=w224, y=w231) -> (x = y?=w230:bool)
                n85 = while {
                  shift-right: [w252] -> w238
                  shift-left: w239 -> [w256]
                  tunnel: w224 -> [w255]
                  tunnel: w237 -> [w254]
                  tunnel: w231 -> [w241]
                  tunnel: w236 -> [w253]
                  tunnel: w235 -> [w246]
                  shift-right: [w251] -> w232
                  shift-left: w234 -> [w250]
                  tunnel: [w246] -> w233
                  tunnel: [w244] -> w228
                  tunnel: [w241] -> w226
                  tunnel: [w240] -> w227
                  tunnel: w225 -> [w242] mode=indexing
                  i -> [w249]
                  stop <- w248 stop-if-true
                  n86 = local read "restart"() -> (w247:i32)
                  n87 = Equal?(x=w247, y=w246) -> (x = y?=w245:bool)
                  n88 = Equal?(x=w249, y=w241) -> (x = y?=w243:bool)
                  n89 = case shown="True" w242 {
                    tunnel: [w257 w264] -> w252
                    tunnel: w256 -> [w257 w271]
                    tunnel: w255 -> [_ w262]
                    tunnel: w249 -> [_ w261]
                    tunnel: w254 -> [_ w263]
                    tunnel: w241 -> [_ w268]
                    tunnel: w253 -> [_ w269]
                    tunnel: [FALSE w266] -> w240
                    tunnel: w250 -> [w258 w267]
                    tunnel: [w258 w265] -> w251
                    frame False {
                      # "jesli false to stop i wygrana bo brak elementow do sprawdzenia"
                    }
                    frame True {
                      n90 = case shown="0" w269 {
                        tunnel: w262 -> [w278 w285 w292]
                        tunnel: w261 -> [w277 w287 w295]
                        tunnel: w268 -> [w275 w284 w291]
                        frame 1, Default {
                          n91 = property on="Cluster 2" class="Clust (strict)"() -> ("Controls[]"=w274:refnum<vi>[])  [unwired: 2 in, 2 out]
                          n92 = Reshape Array(w274, w275, w275) -> (w273:refnum<vi>[][])
                          n93 = Index Array(array=w273, index (row)=w278, index (col)=w277) -> (element=w279:refnum<vi>)
                          n94 = property class="Ctl"(reference=w279, "Disabled"=u8 1, "Visible"=FALSE) -> ()  [unwired: 1 in, 2 out]
                        }
                        frame 2 {
                          n95 = property on="cluster3" class="Clust (strict)"() -> ("Controls[]"=w282:refnum<vi>[])  [unwired: 2 in, 2 out]
                          n96 = Reshape Array(w282, w284, w284) -> (w281:refnum<vi>[][])
                          n97 = Index Array(array=w281, index (row)=w285, index (col)=w287) -> (element=w286:refnum<vi>)
                          n98 = property class="Ctl"(reference=w286, "Disabled"=u8 1, "Visible"=FALSE) -> ()  [unwired: 1 in, 2 out]
                        }
                        frame 0 {
                          n99 = property on="Cluster 1" class="Clust (strict)"() -> ("Controls[]"=w290:refnum<vi>[])  [unwired: 2 in, 2 out]
                          n100 = Reshape Array(w290, w291, w291) -> (w289:refnum<vi>[][])
                          n101 = Index Array(array=w289, index (row)=w292, index (col)=w295) -> (element=w294:refnum<vi>)
                          n102 = property class="Ctl"(reference=w294, "Disabled"=u8 1, "Visible"=FALSE) -> ()  [unwired: 1 in, 2 out]
                        }
                      }
                      n103 = call "licznik.vi"("kolumny"=w261, "wiersze"=w262, "Array"=w263) -> ("licznik"=w260:i32)
                      n104 = Replace Array Subset(array=w271, new element=w260, index (row)=w262, index (col)=w261) -> (w264:i32[][])
                      "licznik" <- w264
                      "obrazy" <- w264
                      n105 = Decrement(x=w267) -> (x-1=w265:i32)
                      n106 = Equal?(x=w260, y=9) -> (x = y?=w266:bool)
                    }
                  }
                  n107 = Or(x=w240, y=w245) -> (x .or. y?=w244:bool)
                  n108 = Or(x=w243, y=w244) -> (x .or. y?=w248:bool)
                }
                n109 = Or(x=w230, y=w228) -> (x .or. y?=w229:bool)
              }
              n110 = case shown="False" w168 {
                tunnel: w167 -> [_ w182]
                tunnel: 0 -> [w180 w190]
                tunnel: [w180 w189] -> w166
                tunnel: w163 -> [_ w185]
                frame False {
                  # "happy face"
                  # "wygrana"
                  "emotikony" <- u16 0 ("Ring")
                }
                frame True {
                  w188 = FALSE
                  # "warunek sprawdzania gry w toku, porownanie ilosci odkrytych pol i min"
                  n111 = local read "miny"() -> (w183:i32[][])
                  n112 = property on="Cluster 1" class="Clust (strict)"("Visible"=w188) -> ()  [unwired: 2 in, 2 out]
                  n113 = property on="cluster3" class="Clust (strict)"("Visible"=w188) -> ()  [unwired: 2 in, 2 out]
                  n114 = property on="Cluster 2" class="Clust (strict)"("Visible"=w188) -> ()  [unwired: 2 in, 2 out]
                  n115 = property on="obrazy" class="Arr (strict)"("Visible"=TRUE) -> ()  [unwired: 2 in, 2 out]
                  n116 = call "trafienie.vi"("miny"=w183, "rozmiar"=w182) -> ("Array 2"=w181:i32[][])  [unwired: 1 in]
                  n117 = Add(x=w181, y=w185) -> (x+y=w184:i32[][])
                  n118 = for {
                    tunnel: w185 -> [w196] mode=indexing
                    tunnel: w181 -> [w195] mode=indexing
                    shift-right: [w192] -> w186
                    shift-left: w184 -> [w194]
                    tunnel: w184 -> [w191] mode=indexing
                    i -> [w193]
                    n119 = for {
                      tunnel: w196 -> [w208] mode=indexing
                      tunnel: w195 -> [w210] mode=indexing
                      tunnel: w193 -> [w198]
                      shift-right: [w199] -> w192
                      shift-left: w194 -> [w211]
                      tunnel: w191 -> [w203] mode=indexing
                      i -> [w197]
                      n120 = Not Equal?(x=w210, y=9) -> (x != y?=w206:bool)
                      n121 = Equal?(x=w203, y=26) -> (x = y?=w201:bool)
                      n122 = Equal?(x=w208, y=17) -> (x = y?=w205:bool)
                      n123 = And(x=w206, y=w205) -> (x .and. y?=w204:bool)
                      n124 = case shown="True" w204 {
                        tunnel: w211 -> [w218 w223]
                        tunnel: w197 -> [_ w222]
                        tunnel: w198 -> [_ w221]
                        tunnel: [w218 w220] -> w200
                        frame False {
                        }
                        frame True {
                          n125 = Replace Array Subset(array=w223, new element=16, index (row)=w221, index (col)=w222) -> (w220:i32[][])
                        }
                      }
                      n126 = case shown="True" w201 {
                        tunnel: w200 -> [w212 w217]
                        tunnel: [w212 w213] -> w199
                        tunnel: w198 -> [_ w216]
                        tunnel: w197 -> [_ w215]
                        frame False {
                        }
                        frame True {
                          n127 = Replace Array Subset(array=w217, new element=17 ("element"), index (row)=w216, index (col)=w215) -> (w213:i32[][])
                        }
                      }
                    }
                  }
                  n128 = Increment(x=w190) -> (x+1=w189:i32)
                  n129 = local write "obrazy"(w186) -> ()
                }
              }
            }
          }
          "restart" <- w60
          "miny" <- w58
          n130 = Equal?(x=w60, y=w64) -> (x = y?=w62:bool)
          n131 = Equal?(x=w66, y=1) -> (x = y?=w63:bool)
          n132 = Or(x=w63, y=w62) -> (x .or. y?=w61:bool)
          "flag" <- w61
        }
        n133 = Get Date/Time In Seconds() -> (seconds since 1Jan1904=w38:timestamp)
        n134 = while {
          tunnel: w38 -> [w52]
          tunnel: w37 -> [_]
          stop <- w54 stop-if-true
          # "obliczanie wyswietlanego czasu na ekranie"
          n135 = Get Date/Time In Seconds() -> (seconds since 1Jan1904=w53:timestamp)
          n136 = Wait Until Next ms Multiple(millisecond multiple=u32 250) -> ()  [unwired: 1 out]
          n137 = Subtract(x=w53, y=w52) -> (x-y=→"czas":dbl)
          n138 = local read "flag"() -> (w54:bool)
        }
        n139 = control-ref of="emotikony"() -> (w36:refnum<vi>)
        n140 = Select(t=w45, s=w39, f=w46) -> (s? t:f=w44:bool)
        n141 = call "koniecgry_zapytanie.vi"("Boolean"=w44, "Ring in"=w36) -> ("T button?"=w40:bool)  [unwired: 9 in]
      }
    }
  }
  n142 = local write "czas"(0.0 ("Tiempo")) -> ()
  n143 = local write "miny"(0 ("Minas")) -> ()
